vi "_Display Calibration Table.vi"(1 "Table Ref":refnum<vi>, 2 "Table Type":u16(ring) items=["Q1 +ve Mass Calibration Table", "Q2 +ve Mass Calibration Table", "Q1 -ve Mass Calibration Table", "Q2 -ve Mass Calibration Table", "Q1 +ve High Resolution Table", "Q2 +ve High Resolution Table", "Q1 +ve Medium Resolution Table", "Q2 +ve Medium Resolution Table", "Q1 +ve Low Resolution Table", "Q2 +ve Low Resolution Table", "Q1 -ve High Resolution Table", "Q2 -ve High Resolution Table", "Q1 -ve Medium Resolution Table", "Q2 -ve Medium Resolution Table", "Q1 -ve Low Resolution Table", "Q2 -ve Low Resolution Table"]) -> ()   [LabVIEW 2012]
uses:
  Configuration/_Global Configuration.vi
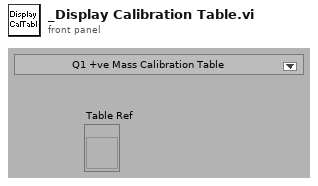
[diagram p1: front panel]
types:
  T1 = cluster{cluster{"Mass":dbl[], "DAC":dbl[]}, string[][]}
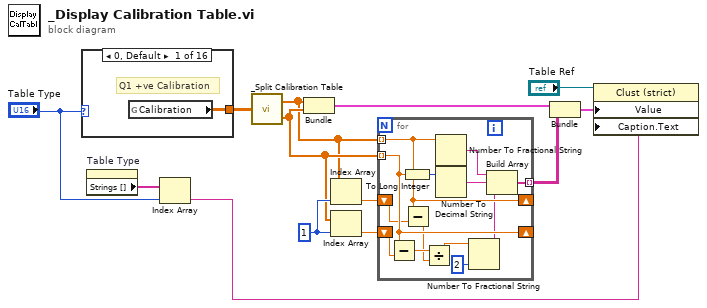
[diagram p0: block diagram]
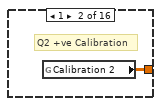
[diagram p2: hidden frame]
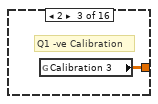
[diagram p3: hidden frame]
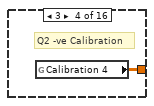
[diagram p4: hidden frame]
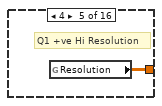
[diagram p5: hidden frame]
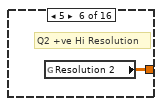
[diagram p6: hidden frame]
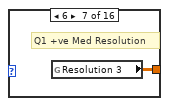
[diagram p7: hidden frame]
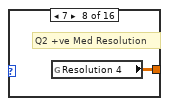
[diagram p8: hidden frame]
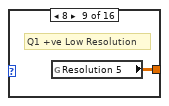
[diagram p9: hidden frame]
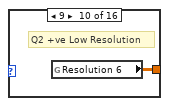
[diagram p10: hidden frame]
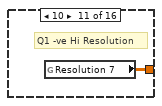
[diagram p11: hidden frame]
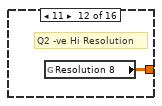
[diagram p12: hidden frame]
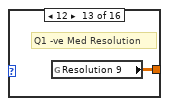
[diagram p13: hidden frame]
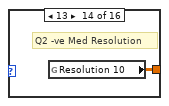
[diagram p14: hidden frame]
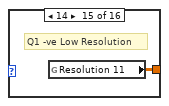
[diagram p15: hidden frame]
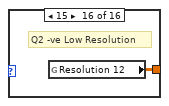
[diagram p16: hidden frame]
diagram:
  w10 = 1 ("index")
  n1 = case shown="0, Default" "Table Type" {
    tunnel: [w14 w15 w16 w17 w18 w19 w20 w21 w22 w23 w24 w25 w26 w27 w28 w29] -> w11
    frame 0, Default {
      # "Q1 +ve Calibration"
      n2 = global read "_Global Configuration.vi" "Calibration"() -> (w14:dbl[][])
    }
    frame 1 {
      # "Q2 +ve Calibration"
      n3 = global read "_Global Configuration.vi" "Calibration 2"() -> (w15:dbl[][])
    }
    frame 2 {
      # "Q1 -ve Calibration"
      n4 = global read "_Global Configuration.vi" "Calibration 3"() -> (w16:dbl[][])
    }
    frame 3 {
      # "Q2 -ve Calibration"
      n5 = global read "_Global Configuration.vi" "Calibration 4"() -> (w17:dbl[][])
    }
    frame 4 {
      # "Q1 +ve Hi Resolution"
      n6 = global read "_Global Configuration.vi" "Resolution"() -> (w18:dbl[][])
    }
    frame 5 {
      # "Q2 +ve Hi Resolution"
      n7 = global read "_Global Configuration.vi" "Resolution 2"() -> (w19:dbl[][])
    }
    frame 6 {
      # "Q1 +ve Med Resolution"
      n8 = global read "_Global Configuration.vi" "Resolution 3"() -> (w20:dbl[][])
    }
    frame 7 {
      # "Q2 +ve Med Resolution"
      n9 = global read "_Global Configuration.vi" "Resolution 4"() -> (w21:dbl[][])
    }
    frame 8 {
      # "Q1 +ve Low Resolution"
      n10 = global read "_Global Configuration.vi" "Resolution 5"() -> (w22:dbl[][])
    }
    frame 9 {
      # "Q2 +ve Low Resolution"
      n11 = global read "_Global Configuration.vi" "Resolution 6"() -> (w23:dbl[][])
    }
    frame 10 {
      # "Q1 -ve Hi Resolution"
      n12 = global read "_Global Configuration.vi" "Resolution 7"() -> (w24:dbl[][])
    }
    frame 11 {
      # "Q2 -ve Hi Resolution"
      n13 = global read "_Global Configuration.vi" "Resolution 8"() -> (w25:dbl[][])
    }
    frame 12 {
      # "Q1 -ve Med Resolution"
      n14 = global read "_Global Configuration.vi" "Resolution 9"() -> (w26:dbl[][])
    }
    frame 13 {
      # "Q2 -ve Med Resolution"
      n15 = global read "_Global Configuration.vi" "Resolution 10"() -> (w27:dbl[][])
    }
    frame 14 {
      # "Q1 -ve Low Resolution"
      n16 = global read "_Global Configuration.vi" "Resolution 11"() -> (w28:dbl[][])
    }
    frame 15 {
      # "Q2 -ve Low Resolution"
      n17 = global read "_Global Configuration.vi" "Resolution 12"() -> (w29:dbl[][])
    }
  }
  n18 = property on="Table Type" class="Ring (strict)"() -> ("Strings []"=w13:string[])  [unwired: 2 in, 2 out]
  n19 = Index Array(array=w13, index="Table Type") -> (element=w1:string)
  n20 = call "_Split Calibration Table.vi"("Calibration"=w11) -> ("Mass"=w8:dbl[], "DAC"=w9:dbl[])
  n21 = Bundle("Mass"=w8, "DAC"=w9) -> (w5:cluster{"Mass":dbl[], "DAC":dbl[]})  [unwired: 1 out]
  n22 = Index Array(array=w8, index=w10) -> (element=w7:dbl)
  n23 = Index Array(array=w9, index=w10) -> (element=w6:dbl)
  n24 = for {
    tunnel: [w39] -> w4 mode=indexing
    tunnel: w8 -> [w36] mode=indexing
    tunnel: w9 -> [w38] mode=indexing
    shift-right: [w36] -> _
    shift-left: w7 -> [w35]
    shift-right: [w38] -> _
    shift-left: w6 -> [w37]
    n25 = Subtract(x=w38, y=w37) -> (x-y=w34:dbl)
    n26 = To Long Integer(number=w38) -> (32bit integer=w42:i32)
    n27 = Subtract(x=w36, y=w35) -> (x-y=w33:dbl)
    n28 = Divide(x=w34, y=w33) -> (x/y=w32:dbl)
    n29 = Number To Fractional String(number=w36) -> (F-format string=w41:string)  [unwired: 3 out]
    n30 = Number To Decimal String(number=w42) -> (decimal integer string=w40:string)  [unwired: 1 out]
    n31 = Number To Fractional String(number=w32, precision (6)=i16 2) -> (F-format string=w30:string)  [unwired: 2 out]
    n32 = Build Array(w41, w40, w30) -> (w39:string[])
  }
  n33 = Bundle(w5, w4) -> (w2:T1)  [unwired: 1 out]
  n34 = property class="Clust (strict)"(reference="Table Ref", "Value"=w2, "Caption.Text"=w1) -> ()  [unwired: 1 in, 2 out]
